vi "Create RxTx.vi"(8 "error in (no error)":errorcluster, 10 "Remote IP":string="200.131.64.49", 11 "Roda_Filtros in":refnum<class "Roda_Filtros.lvclass">) -> (0 "error out":errorcluster, 3 "Roda_Filtros out":refnum<class "Roda_Filtros.lvclass">)   [LabVIEW 2018, in "Roda_Filtros.lvclass"]
uses:
  Roda_Filtros.lvclass
  Roda_Filtros.lvclass/Roda_Filtros.ctl
  RxTx/RxTx.lvclass
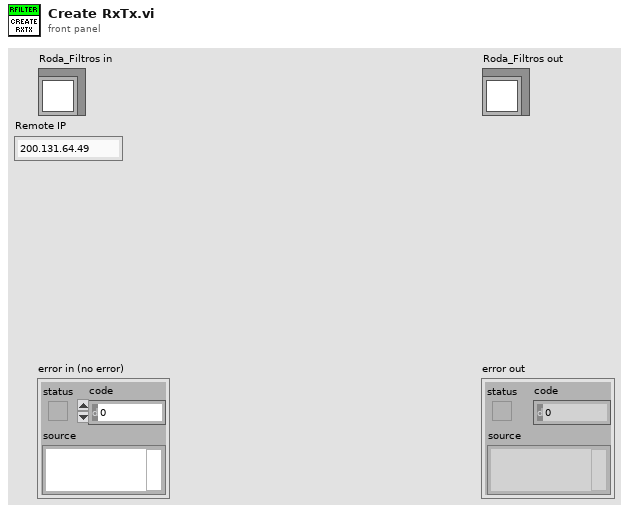
[diagram p1: front panel]
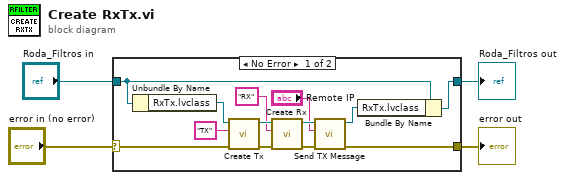
[diagram p0: block diagram]
diagram:
  n1 = case shown="No Error" "error in (no error)" {
    selector: "error in (no error)" -> [w13 w19]
    tunnel: [w7 w19] -> w3
    tunnel: [w16 w18] -> w1
    tunnel: "Roda_Filtros in" -> [w17 w18]
    frame No Error {
      n2 = Unbundle By Name(w17) -> ("RxTx.lvclass"=w12:refnum<class "RxTx.lvclass">)
      n3 = call "Create Tx.vi"("error in (no error)"=w13, "Writer Name"="TX", "RxTx in"=w12) -> ("error out"=w14:errorcluster, "RxTx out"=w15:refnum<class "RxTx.lvclass">)  [unwired: 7 in]
      n4 = call "Create Rx.vi"("error in (no error)"=w14, "Reader Name"="RX", "RxTx in"=w15) -> ("error out"=w6:errorcluster, "RxTx out"=w9:refnum<class "RxTx.lvclass">)  [unwired: 7 in]
      n5 = call "Send TX Message.vi"("error in (no error)"=w6, "element"="Remote IP", "RxTx in"=w9) -> ("error out"=w7:errorcluster, "RxTx out"=w8:refnum<class "RxTx.lvclass">)  [unwired: 7 in]
      n6 = Bundle By Name(cluster=w17, "RxTx.lvclass"=w8) -> (w16:refnum<class "Roda_Filtros.lvclass">)
    }
    frame Error {
    }
  }
  "error out" <- w3
  "Roda_Filtros out" <- w1
